vi "vertragen_versnellen_Deel2 (SubVI).vi"(9 "rechtermotor":dbl, 10 "linker motor":dbl) -> (1 "rechtermotor na":dbl, 2 "linker motor na":dbl)   [LabVIEW 2019]
uses:
  <vilib>/myRIO/Common/Instrument Driver Framework/Utilities/typedefs/Generic FPGA Reference.ctl
  <vilib>/myRIO/Common/Instrument Driver Framework/Utilities/typedefs/myRIO v1.0 Reference.ctl
  <vilib>/myRIO/Common/Instrument Driver Framework/Utilities/typedefs/Hardware Version Enum.ctl
  <vilib>/myRIO/Common/Instrument Driver Framework/Utilities/typedefs/myRIO Generic Hardware Reference.ctl
  <vilib>/myRIO/Common/Instrument Driver Framework/Utilities/vis/Is FPGA Ref Available.vi
  <vilib>/userDefined/High Color/nirio_resource_hc.ctl
  <vilib>/myRIO/Express VI/Onboard IO/AI/AI Express VI.xnode
  <vilib>/myRIO/Instrument Drivers/Onboard IO/AI/vis/Read.vi
  <vilib>/myRIO/Instrument Drivers/Onboard IO/AI/AI.lvlib
  <vilib>/myRIO/Common/Instrument Driver Framework/Utilities/typedefs/Analog Scaling Constants.ctl
  <vilib>/myRIO/Common/Instrument Driver Framework/Utilities/typedefs/Analog Scaling Constants List.ctl
  <vilib>/myRIO/Common/Instrument Driver Framework/myRIO v1.0/AI/typedefs/AI Channels Enum.ctl
  <vilib>/myRIO/Common/Instrument Driver Framework/myRIO v1.0/AI/typedefs/AI Channels List.ctl
  <vilib>/myRIO/Instrument Drivers/Onboard IO/AI/typedefs/AI Reference.ctl
  <vilib>/myRIO/Instrument Drivers/Onboard IO/AI/vis/myRIO AI Open.xnode
  <vilib>/myRIO/Common/Instrument Driver Framework/myRIO v1.0/AI/vis/myRIO v1.1 Open AI.vi
panel:
  out "A/AI3 (Pin 9)":dbl
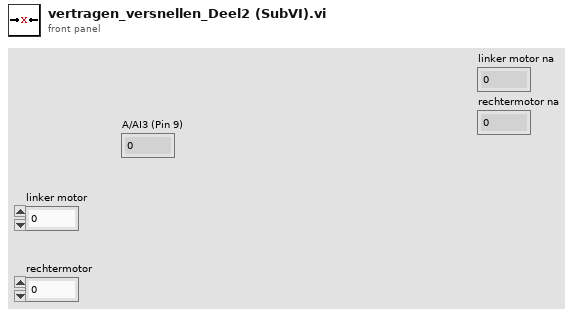
[diagram p1: front panel]
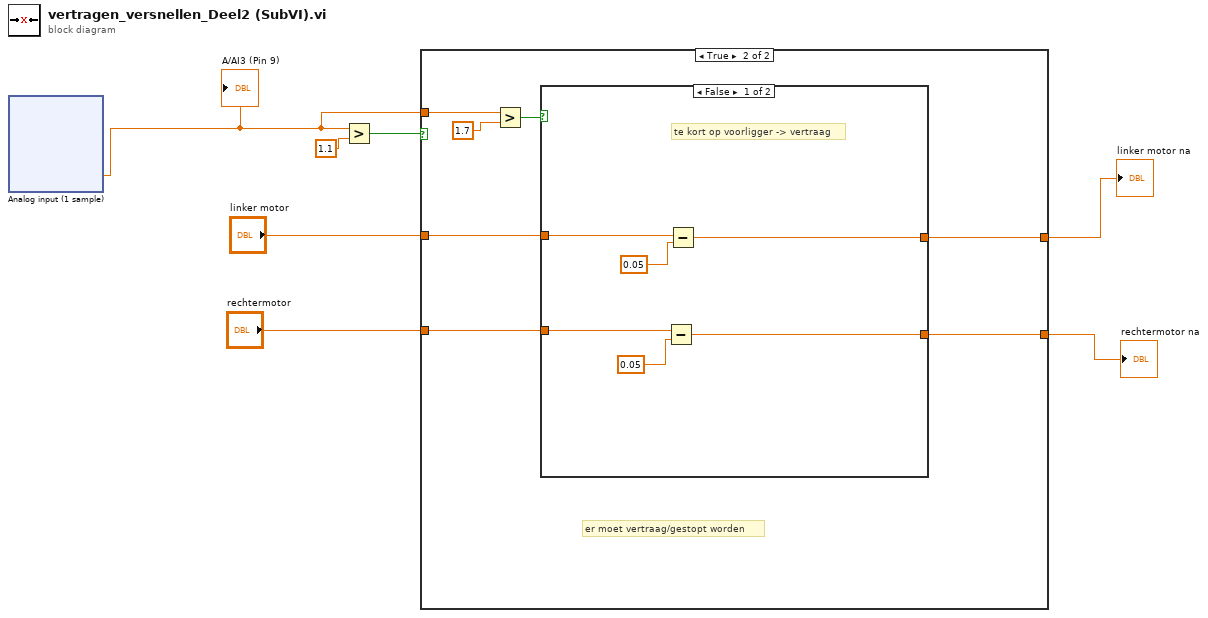
[diagram p0: block diagram]
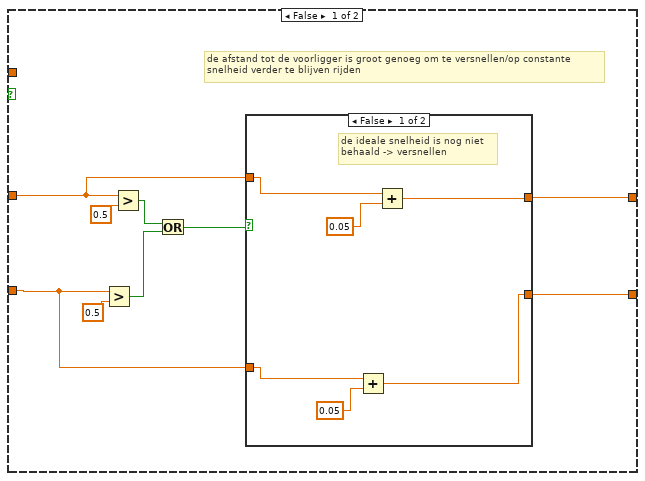
[diagram p2: hidden frame]
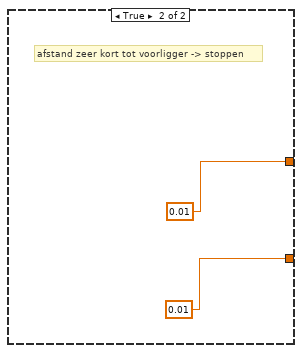
[diagram p4: hidden frame]
diagram:
  n1 = xnode "Analog input (1 sample)"() -> ("A/AI3 (Pin 9)"=w2:dbl)  [unwired: 1 in, 1 out]
  "A/AI3 (Pin 9)" <- w2
  n2 = Greater?(x=w2, y=1.1) -> (0:w6:bool)
  n3 = case shown="True" w6 {
    tunnel: w2 -> [_ w30]
    tunnel: "linker motor" -> [w11 w28]
    tunnel: "rechtermotor" -> [w10 w27]
    tunnel: [w9 w26] -> w1
    tunnel: [w8 w25] -> w3
    frame False {
      # "de afstand tot de voorligger is groot genoeg om te versnellen/op constante\nsnelheid verder te blijven rijden"
      n4 = Greater?(x=w10, y=0.5) -> (0:w13:bool)
      n5 = Greater?(x=w11, y=0.5) -> (0:w14:bool)
      n6 = Or(x=w14, y=w13) -> (x .or. y?=w12:bool)
      n7 = case shown="False" w12 {
        tunnel: w11 -> [w22 w24]
        tunnel: w10 -> [w19 w23]
        tunnel: [w21 w24] -> w9
        tunnel: [w17 w23] -> w8
        frame False {
          # "de ideale snelheid is nog niet \nbehaald -> versnellen"
          n8 = Add(x=w19, y=0.05) -> (x+y=w17:dbl)
          n9 = Add(x=w22, y=0.05) -> (x+y=w21:dbl)
        }
        frame True {
          # "de ideale snelheid is al behaald"
        }
      }
    }
    frame True {
      # "er moet vertraag/gestopt worden"
      n10 = Greater?(x=w30, y=1.7) -> (0:w29:bool)
      n11 = case shown="False" w29 {
        tunnel: w28 -> [w37 _]
        tunnel: w27 -> [w35 _]
        tunnel: [w33 0.01] -> w25
        tunnel: [w32 0.01] -> w26
        frame False {
          # "te kort op voorligger -> vertraag"
          n12 = Subtract(x=w35, y=0.05) -> (x-y=w33:dbl)
          n13 = Subtract(x=w37, y=0.05) -> (x-y=w32:dbl)
        }
        frame True {
          # "afstand zeer kort tot voorligger -> stoppen"
        }
      }
    }
  }
  "linker motor na" <- w1
  "rechtermotor na" <- w3
